vi "_Read.vi"(8 "error in (no error)":errorcluster, 11 "Wavelength Meter in":refnum<class "Wavelength Meter.lvclass">) -> (0 "error out":errorcluster, 2 "4 Data Points":dbl[](array[numeric]), 3 "Wavelength Meter out":refnum<class "Wavelength Meter.lvclass">)   [LabVIEW 2009, in "Wavelength Meter.lvclass"]
uses:
  Wavelength Meter.lvclass
  Utility Classes/Readable/Readable.lvclass
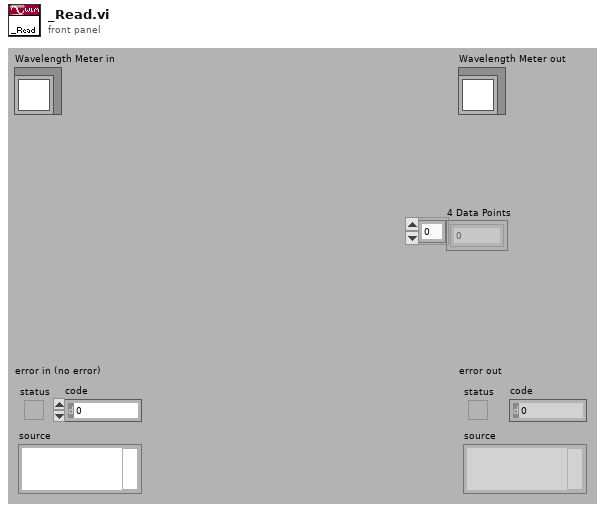
[diagram p1: front panel]
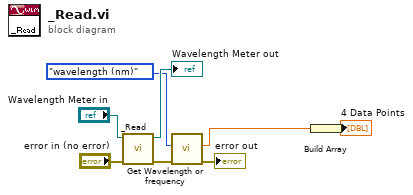
[diagram p0: block diagram]
diagram:
  n1 = call-parent "_Read.vi"("error in (no error)"="error in (no error)", "Readable in"="Wavelength Meter in") -> ("error out"=w5:errorcluster, "Readable out"=→"Wavelength Meter out":refnum<class "Wavelength Meter.lvclass">)  [unwired: 8 out]
  n2 = call "Get Wavelength or frequency.vi"("error in (no error)"=w5, "mode (wavelength)"=enum16{"wavelength (nm)", "frequency (THz)"}."wavelength (nm)") -> ("error out"=→"error out":errorcluster, "result"=w2:dbl)  [unwired: 1 in, 7 out]
  n3 = Build Array(w2) -> (→"4 Data Points":dbl[])
